vi "Generate Single Chirp.vi"(10 "User Specified":T1={"Hardware Configuration"={"Signal Channel"="PXI1Slot7/ao0", "Response Channel"="PXI1Slot7/ai0", "Trigger Channel"="/PXI1Slot7/PFI0", "Number of Acquisitions"=1.0}, "Analysis Configuration"={"Statistics"=TRUE}, "Signal Type"=enum."From Excel", "New Data Behavior"=enum."Replace", "Signal Configuration"={"Chirp Amplitude"=0.0, "I/O Limit"=0.0, "Sample Rate"=0.0, "Chirp Duration (s)"=0.0, "Upper Frequency"=0.0, "Lower Frequency"=0.0, "Windowing"=enum."None"}, "Waveform File"="", "Save Location"=""}) -> (0 "error out":errorcluster, 1 "dt":dbl, 2 "Number of samples":dbl, 3 "Chirp":waveform(dbl)(graph))   [LabVIEW 2017]
uses:
  controls/User Specified Data.ctl
  controls/HW Configuration.ctl
  controls/Analysis Configuration.ctl
  controls/New Data Behavior.ctl
  controls/Signal Configuration.ctl
  <vilib>/Analysis/4window.llb/Cosine Tapered Window (DBL).vi
  <vilib>/Analysis/4window.llb/Flat Top Window (DBL).vi
  <vilib>/Analysis/4window.llb/Hamming Window (DBL).vi
  <vilib>/Analysis/4window.llb/Hanning Window (DBL).vi
  <vilib>/Analysis/4window.llb/Kaiser-Bessel Window (DBL).vi
  <vilib>/Analysis/4window.llb/Force Window (DBL).vi
  <vilib>/Analysis/4window.llb/AllCosWindow (DBL).vi
  <vilib>/express/express analysis/Spectral/Block/exnSpectralBlock spectral measurements power poly.vi
  <vilib>/express/express analysis/Spectral/Block/exnSpectralBlock spectral measurements power WFM.vi
  <vilib>/ErrorRing/Error Ring.xnode
  <vilib>/express/express analysis/Spectral/XNode/ExpressSpectralMeasurementsBlockNode.xnode
  <vilib>/Analysis/NI_AALPro.lvlib
  <vilib>/Analysis/NI_AALBase.lvlib
panel:
  out "Unwindowed Chirp":waveform(dbl)(graph)
  out "Unwindowed FFT":cluster{"f0":dbl, "df":dbl, "magnitude":dbl[]}(graph)
  out "Windowed FFT":cluster{"f0":dbl, "df":dbl, "magnitude":dbl[]}(graph)
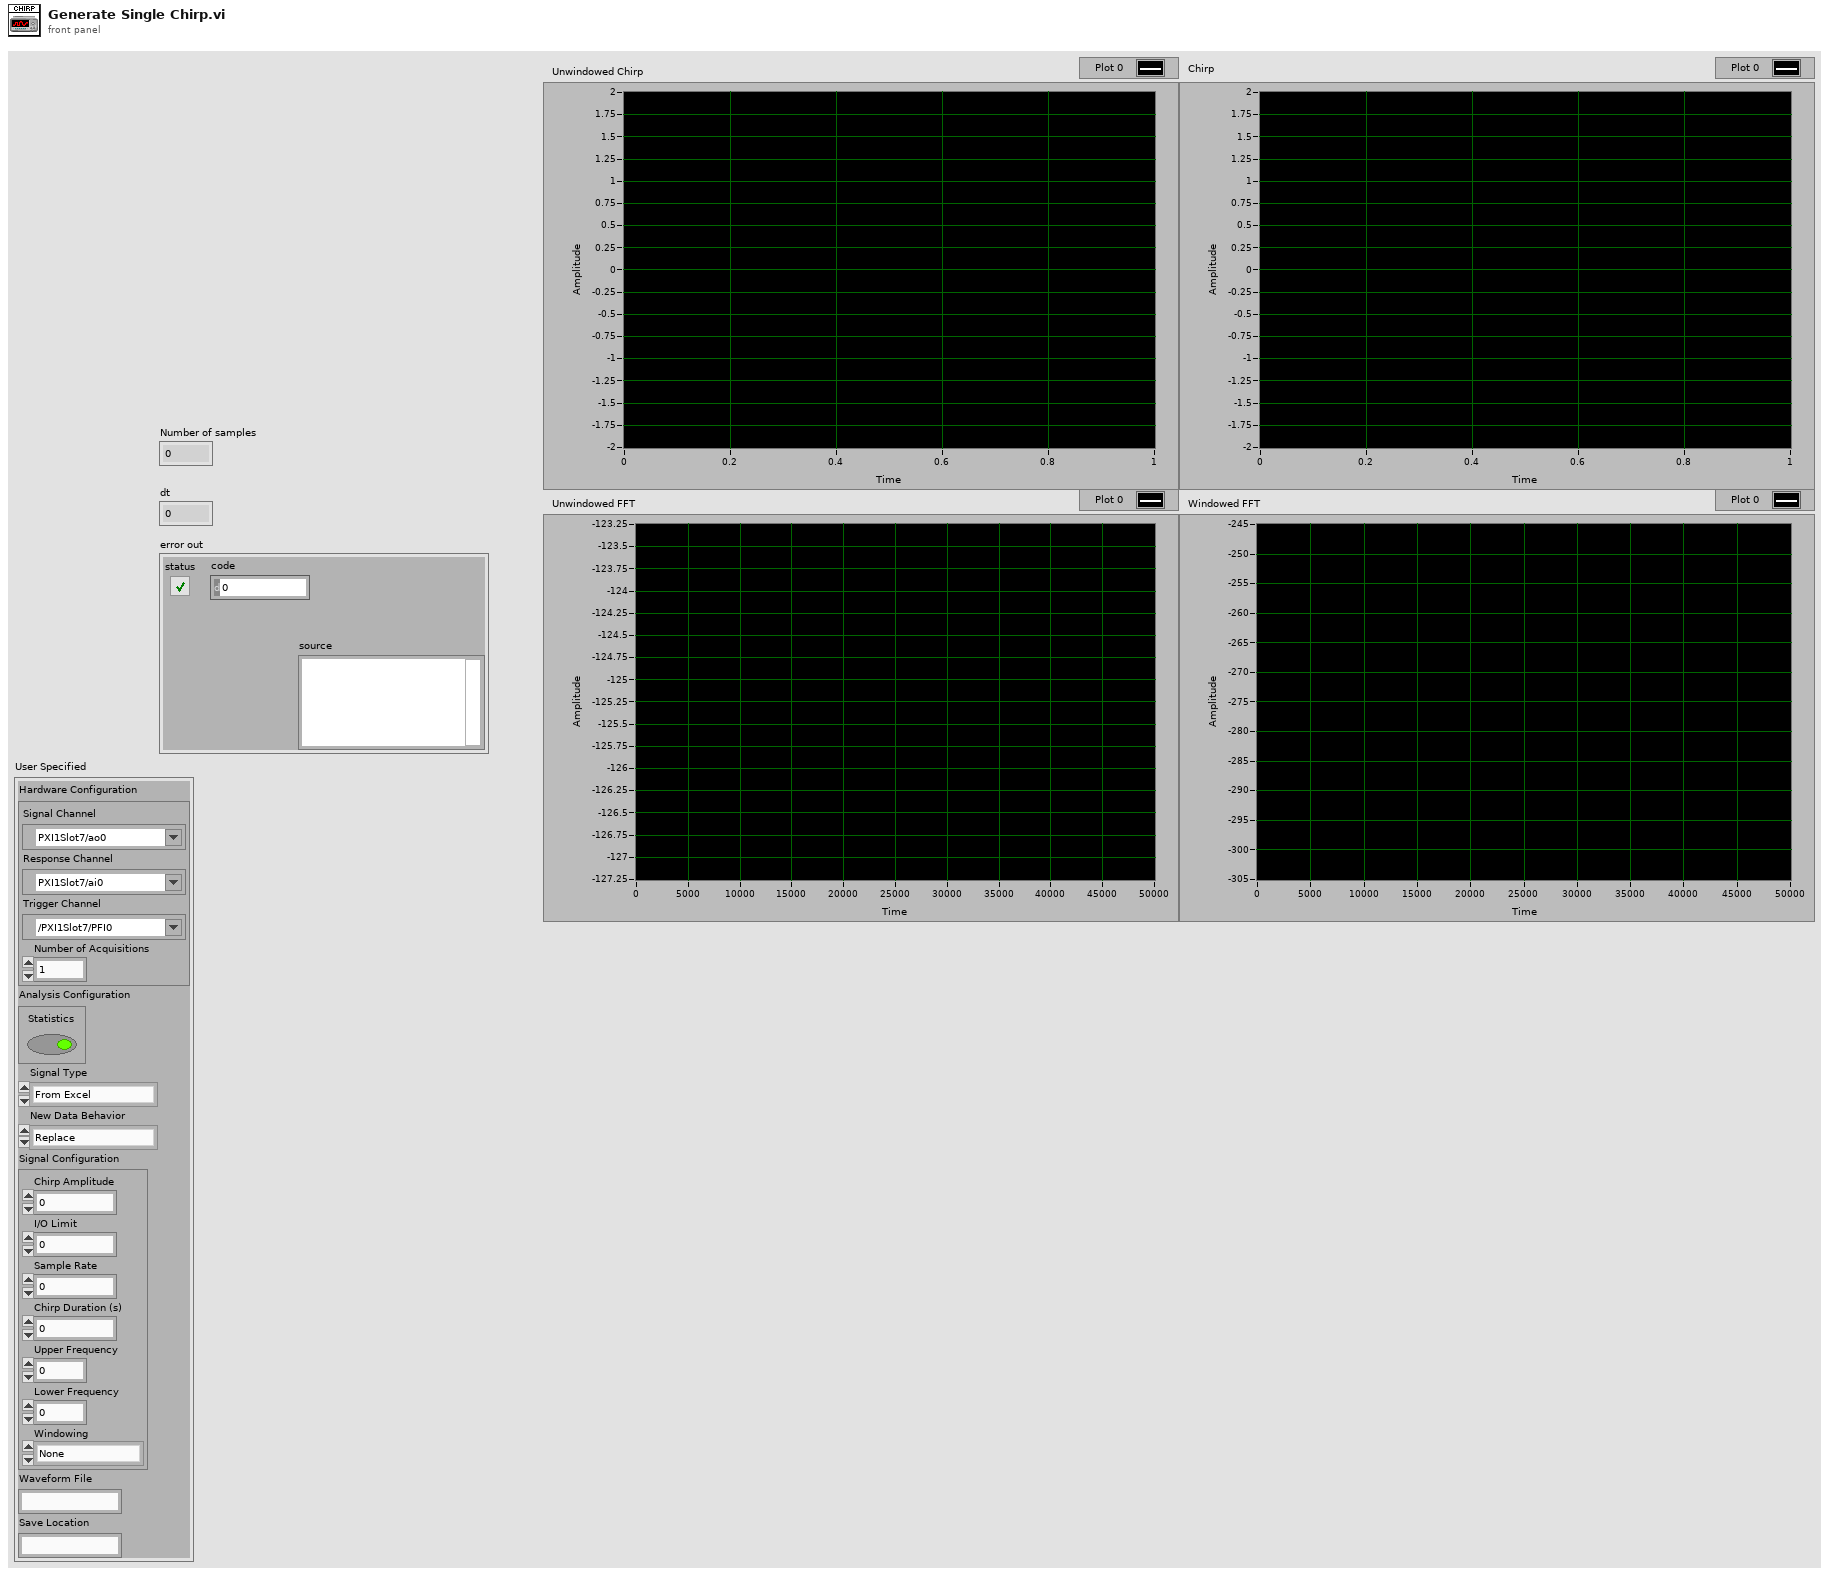
[diagram p1: front panel]
types:
  T1 = typedef "User Specified Data.ctl" = cluster{"Hardware Configuration":T2, "Analysis Configuration":T3, "Signal Type":enum16{"From Excel", "Single Chirp"}, "New Data Behavior":T4, "Signal Configuration":T5, "Waveform File":string, "Save Location":string}
  T2 = typedef "HW Configuration.ctl" = cluster{"Signal Channel":tag, "Response Channel":tag, "Trigger Channel":tag, "Number of Acquisitions":dbl}
  T3 = typedef "Analysis Configuration.ctl" = cluster{"Statistics":bool}
  T4 = typedef "New Data Behavior.ctl" = enum16{"Replace", "Overlay", "Append"}
  T5 = typedef "Signal Configuration.ctl" = cluster{"Chirp Amplitude":dbl, "I/O Limit":dbl, "Sample Rate":dbl, "Chirp Duration (s)":dbl, "Upper Frequency":dbl, "Lower Frequency":dbl, "Windowing":enum16{"None", "Exponential", "Flat top", "Hamming", "Hanning", "Kaiser-Bessel", "Rectangular"}}
  T6 = enum16{"None", "Exponential", "Flat top", "Hamming", "Hanning", "Kaiser-Bessel", "Rectangular"}
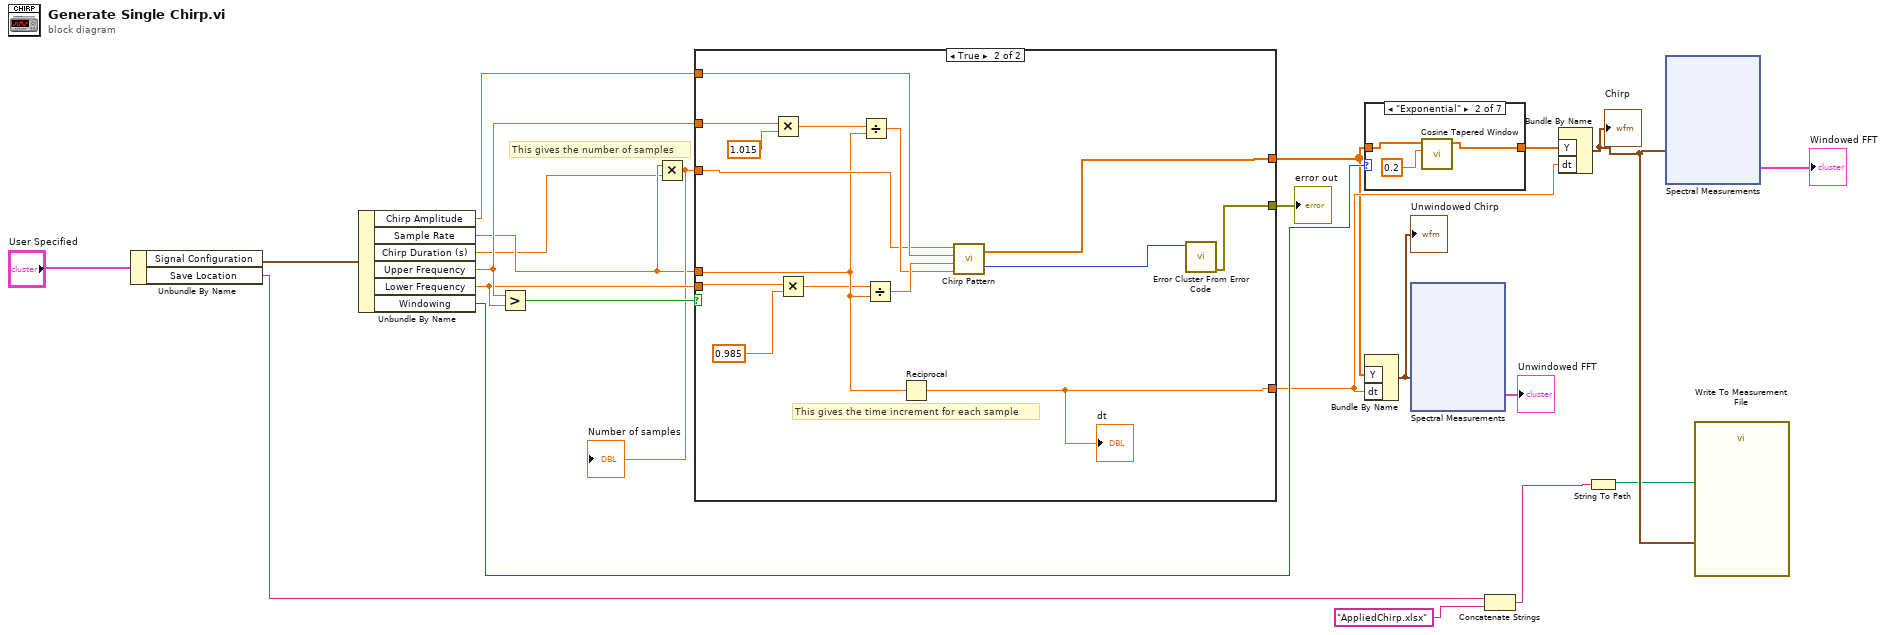
[diagram p0: block diagram]
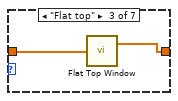
[diagram p3: hidden frame]
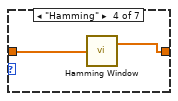
[diagram p4: hidden frame]
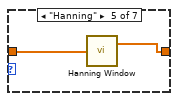
[diagram p5: hidden frame]
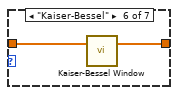
[diagram p6: hidden frame]
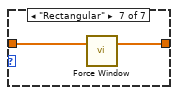
[diagram p7: hidden frame]
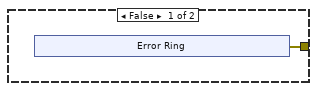
[diagram p8: hidden frame]
diagram:
  # "This gives the number of samples"
  n1 = Unbundle By Name("User Specified") -> ("Signal Configuration"=w7:T5, "Save Location"=w5:string)
  n2 = Unbundle By Name(w7) -> ("Chirp Amplitude"=w20:dbl, "Sample Rate"=w9:dbl, "Chirp Duration (s)"=w8:dbl, "Upper Frequency"=w19:dbl, "Lower Frequency"=w18:dbl, "Windowing"=w17:T6)
  n3 = Greater?(x=w19, y=w18) -> (0:w22:bool)
  n4 = Multiply(x=w9, y=w8) -> (x*y=w10:dbl)
  "Number of samples" <- w10
  n5 = case shown="True" w22 {
    tunnel: w19 -> [_ w31]
    tunnel: w18 -> [_ w33]
    tunnel: [w23 w36] -> w21
    tunnel: w9 -> [_ w39]
    tunnel: w10 -> [_ w40]
    tunnel: w20 -> [_ w41]
    tunnel: [_ w38] -> w12
    tunnel: [_ w35] -> w13
    frame False {
      n6 = xnode "Error Ring"() -> ("error out"=w23:errorcluster)
    }
    frame True {
      # "This gives the time increment for each sample"
      n7 = Multiply(x=w31, y=1.015) -> (x*y=w30:dbl)
      n8 = Multiply(x=w33, y=0.985) -> (x*y=w32:dbl)
      n9 = Divide(x=w30, y=w39) -> (x/y=w42:dbl)
      n10 = Divide(x=w32, y=w39) -> (x/y=w43:dbl)
      n11 = Reciprocal(x=w39) -> (1/x=w35:dbl)
      "dt" <- w35
      n12 = call <vilib>:"Chirp Pattern.vi"("f2"=w42, "f1"=w43, "amplitude"=w41, "samples"=w40) -> ("error"=w37:i32, "Chirp Pattern"=w38:dbl[])
      n13 = call <vilib>:"Error Cluster From Error Code.vi"("error code (0)"=w37) -> ("error out"=w36:errorcluster)  [unwired: 8 in]
    }
  }
  "error out" <- w21
  n14 = case shown="\"Exponential\"" w17 {
    tunnel: [w44 w46 w48 w51 w53 w55 w56] -> w16
    tunnel: w12 -> [w44 w47 w49 w50 w52 w54 w57]
    frame "None", Default {
    }
    frame "Exponential" {
      n15 = call-poly <vilib>:"Cosine Tapered Window.vi"("ratio"=0.2, "X"=w47) -> ("Windowed X"=w46:dbl[])  [unwired: 8 in, 1 out]
    }
    frame "Flat top" {
      n16 = call-poly <vilib>:"Flat Top Window.vi"("X"=w49) -> ("Windowed X"=w48:dbl[])  [unwired: 1 out]
    }
    frame "Hamming" {
      n17 = call-poly <vilib>:"Hamming Window.vi"("X"=w50) -> ("Windowed X"=w51:dbl[])  [unwired: 1 out]
    }
    frame "Hanning" {
      n18 = call-poly <vilib>:"Hanning Window.vi"("X"=w52) -> ("Windowed X"=w53:dbl[])  [unwired: 1 out]
    }
    frame "Kaiser-Bessel" {
      n19 = call-poly <vilib>:"Kaiser-Bessel Window.vi"("X"=w54) -> ("Windowed X"=w55:dbl[])  [unwired: 1 in, 1 out]
    }
    frame "Rectangular" {
      n20 = call-poly <vilib>:"Force Window.vi"("X"=w57) -> ("Windowed X"=w56:dbl[])  [unwired: 1 in, 1 out]
    }
  }
  n21 = Bundle By Name("Y"=w12, "dt"=w13) -> (w11:waveform(dbl))  [unwired: 1 in]
  "Unwindowed Chirp" <- w11
  n22 = xnode "Spectral Measurements"("Signals"=w11) -> ("Power Spectrum"=→"Unwindowed FFT":cluster{"f0":dbl, "df":dbl, "magnitude":dbl[]})  [unwired: 1 in, 1 out]
  n23 = Concatenate Strings(w5, "AppliedChirp.xlsx") -> (w3:string)
  n24 = Bundle By Name("Y"=w16, "dt"=w13) -> (w6:waveform(dbl))  [unwired: 1 in]
  "Chirp" <- w6
  n25 = String To Path(string=w3) -> (path=w2:path)
  n26 = xnode "Spectral Measurements"("Signals"=w6) -> ("Power Spectrum"=→"Windowed FFT":cluster{"f0":dbl, "df":dbl, "magnitude":dbl[]})  [unwired: 1 in, 1 out]
  n27 = call "Write To Measurement File"("Signals"=w6, "Filename"=w2) -> ()  [unwired: 15 in, 3 out]
